vi "AutonControl.vi"(7 "Disabled":bool=TRUE, 8 "error in":errorcluster, 9 "Gamepad Data":T1, 10 "HMI to Control":T2, 11 "SensorInputData":T6) -> (0 "error out":errorcluster, 2 "HMI to Control Out":T2, 3 "SensorInputDataOut":T6)   [LabVIEW 2014]
uses:
  Typedefs/SensorInputData.ctl
  Typedefs/HMI_to_Control.ctl
  Typedefs/Arm States.ctl
  Typedefs/ClawStates.ctl
  Typedefs/IntakeWheelSenseOrManual.ctl
  Typedefs/GamepadData.ctl
  scriptlib/auto_data.vi
panel:
  out "autontime":i32
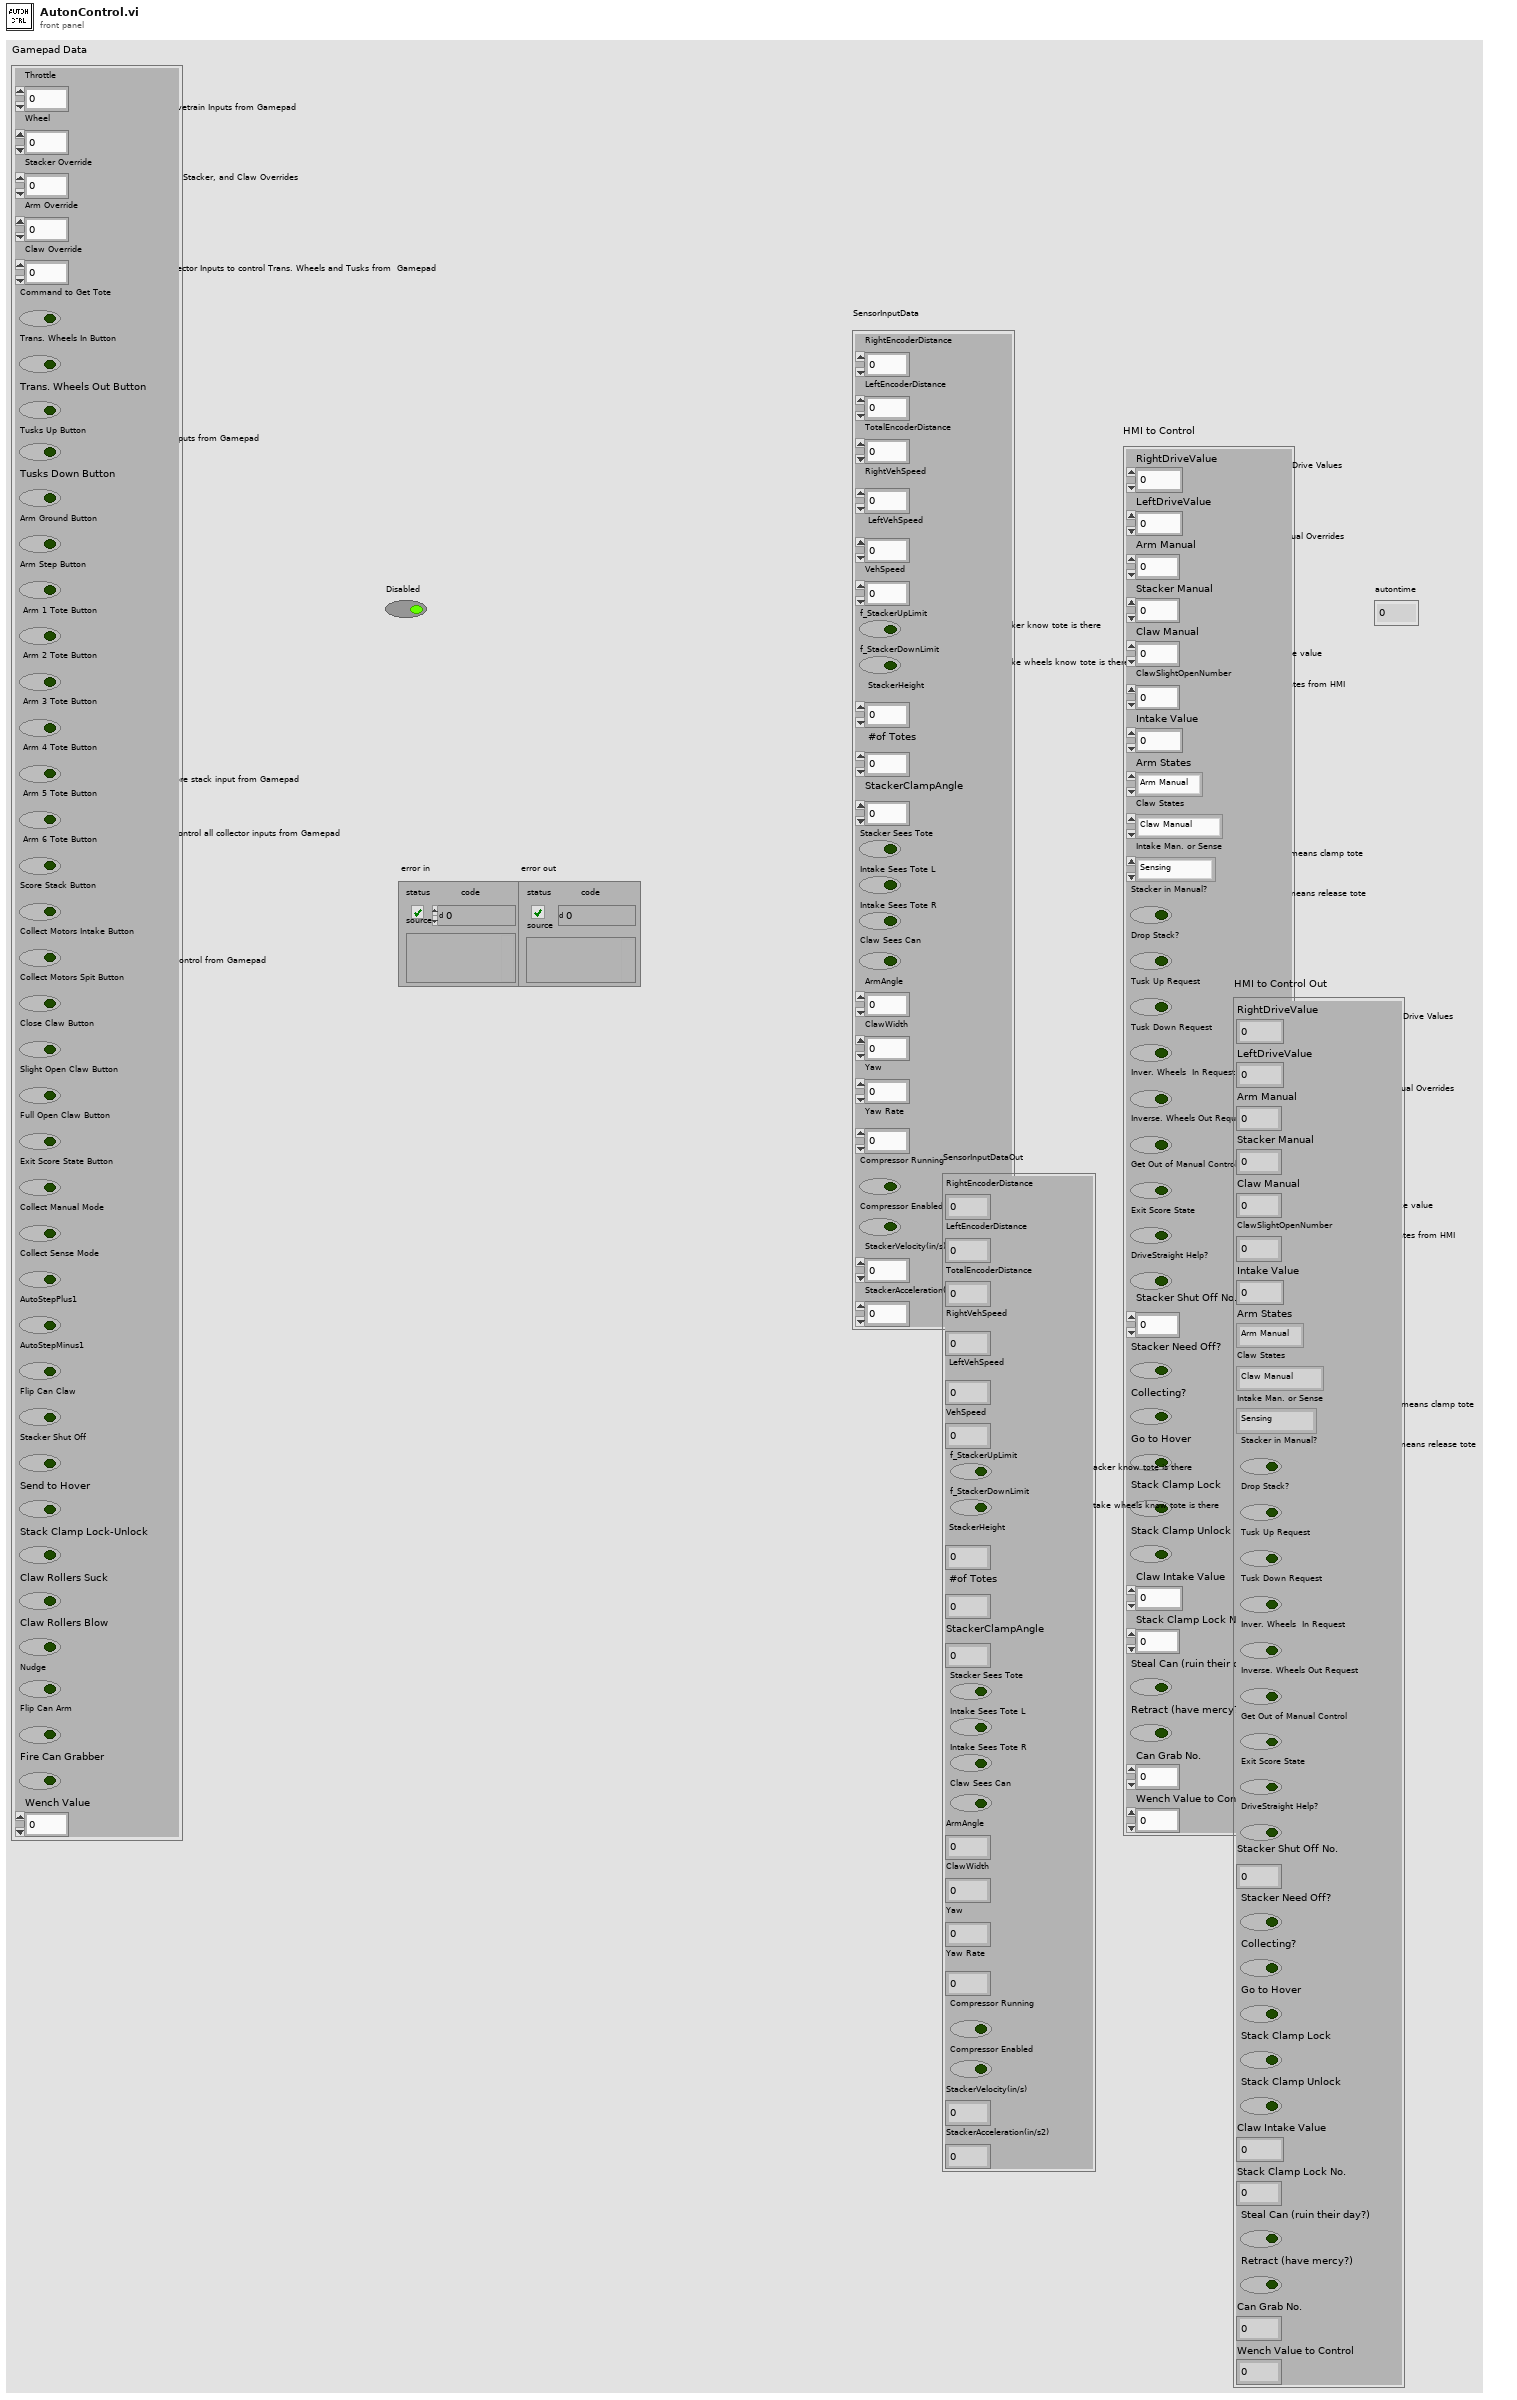
[diagram p1: front panel]
types:
  T1 = typedef "GamepadData.ctl" = cluster{"Throttle":dbl, "Wheel":dbl, "Stacker Override":dbl, "Arm Override ":dbl, "Claw Override":dbl, "Command to Get Tote":bool, "Trans. Wheels In Button":bool, "Trans. Wheels Out Button":bool, "Tusks Up Button":bool, "Tusks Down Button":bool, "Arm Ground Button":bool, "Arm Step Button":bool, " Arm 1 Tote Button":bool, " Arm 2 Tote Button":bool, " Arm 3 Tote Button ":bool, " Arm 4 Tote Button":bool, " Arm 5 Tote Button":bool, " Arm 6 Tote Button":bool, "Score Stack Button":bool, "Collect Motors Intake Button":bool, "Collect Motors Spit Button":bool, "Close Claw Button":bool, "Slight Open Claw Button":bool, "Full Open Claw Button ":bool, "Exit Score State Button":bool, "Collect Manual Mode ":bool, "Collect Sense Mode":bool, "AutoStepPlus1":bool, "AutoStepMinus1":bool, "Flip Can Claw":bool, "Stacker Shut Off":bool, "Send to Hover ":bool, "Stack Clamp Lock-Unlock ":bool, "Claw Rollers Suck ":bool, "Claw Rollers Blow ":bool, "Nudge":bool, "Flip Can Arm ":bool, "Fire Can Grabber":bool, "Wench Value":dbl}
  T2 = typedef "HMI_to_Control.ctl" = cluster{"RightDriveValue":dbl, "LeftDriveValue":dbl, "Arm Manual ":dbl, "Stacker Manual ":dbl, "Claw Manual ":dbl, "ClawSlightOpenNumber":i8, "Intake Value ":sgl, "Arm States":T3, "Claw States":T4, "Intake Man. or Sense":T5, "Stacker in Manual?":bool, "Drop Stack? ":bool, "Tusk Up Request":bool, "Tusk Down Request":bool, "Inver. Wheels  In Request":bool, "Inverse. Wheels Out Request ":bool, "Get Out of Manual Control":bool, "Exit Score State":bool, "DriveStraight Help?":bool, "Stacker Shut Off No.":i8, "Stacker Need Off?":bool, "Collecting?":bool, "Go to Hover":bool, "Stack Clamp Lock ":bool, "Stack Clamp Unlock ":bool, "Claw Intake Value ":sgl, "Stack Clamp Lock No. ":i8, "Steal Can (ruin their day?)":bool, "Retract (have mercy?)":bool, "Can Grab No. ":i8, "Wench Value to Control ":dbl}
  T3 = typedef "Arm States.ctl" = enum16{"Arm Manual ", "Ground", "Step", "1 Tote", "2 Tote", "3 Tote", "4 Tote", "5 Tote", "6 Tote", "Flip Can Arm", "Grab Can in auto", "Nudge"}
  T4 = typedef "ClawStates.ctl" = enum16{"Claw Manual ", "Claw Open", "Claw Closed", "Claw Slight Open", "Flip Can"}
  T5 = typedef "IntakeWheelSenseOrManual.ctl" = enum16{"Sensing", "Manual "}
  T6 = typedef "SensorInputData.ctl" = cluster{"RightEncoderDistance":dbl, "LeftEncoderDistance":dbl, "TotalEncoderDistance":dbl, "RightVehSpeed":dbl, "LeftVehSpeed":dbl, "VehSpeed":dbl, "f_StackerUpLimit":bool, "f_StackerDownLimit":bool, "StackerHeight":dbl, "#of Totes":u8, "StackerClampAngle":dbl, "Stacker Sees Tote":bool, "Intake Sees Tote L":bool, "Intake Sees Tote R":bool, "Claw Sees Can":bool, "ArmAngle":dbl, "ClawWidth":dbl, "Yaw":dbl, "Yaw Rate":dbl, "Compressor Running":bool, "Compressor Enabled":bool, "StackerVelocity(in/s)":dbl, "StackerAcceleration(in/s2)":dbl}
  T7 = typedef "vi_execute.ctl" = cluster{"arguments":string[], "command":string, "refnum valid check":bool, "vi_ind":u8}
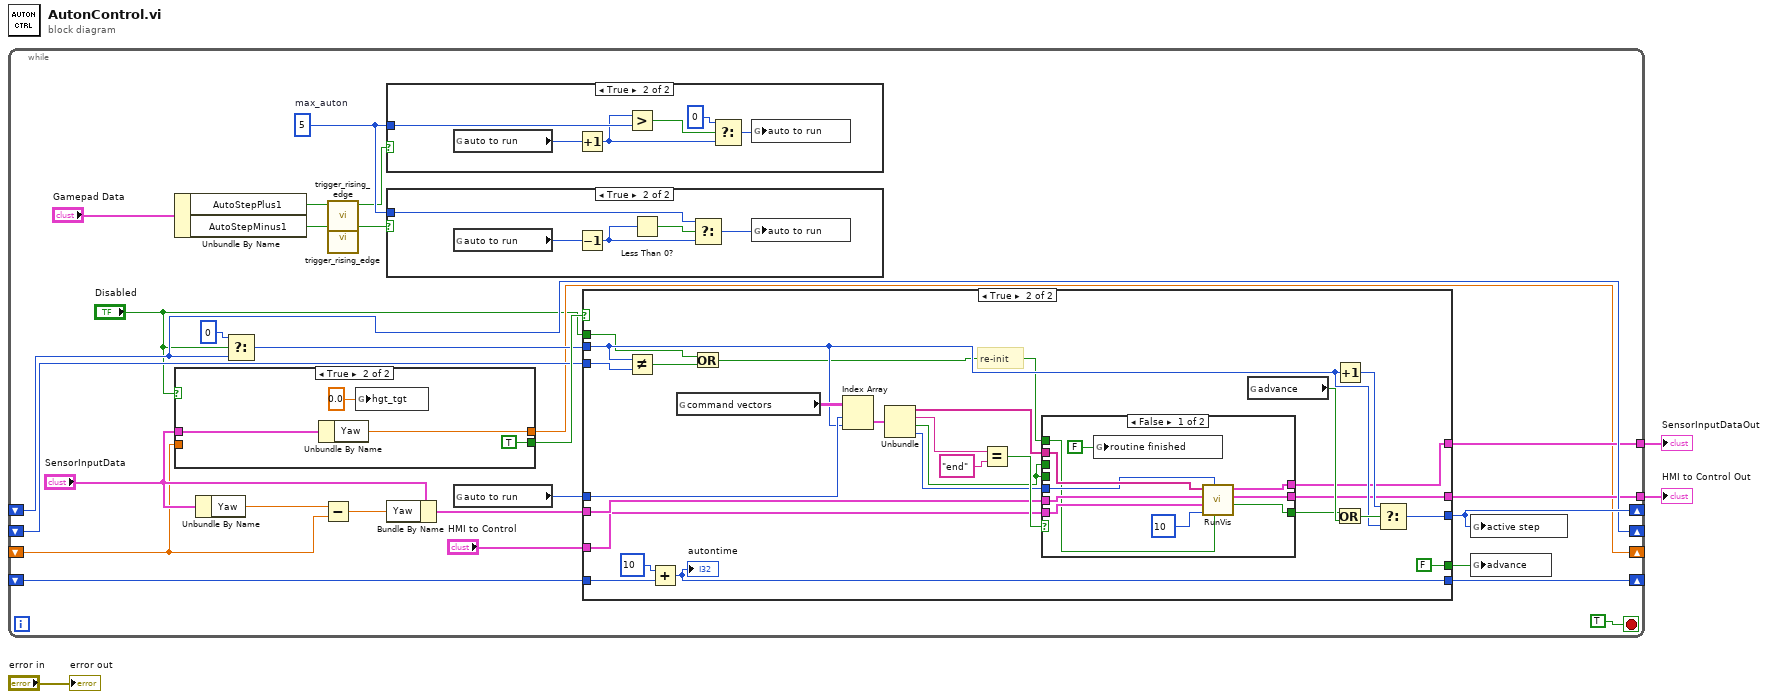
[diagram p0: block diagram]
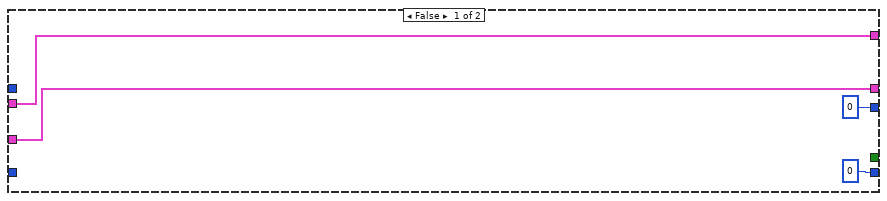
[diagram p4: hidden frame]
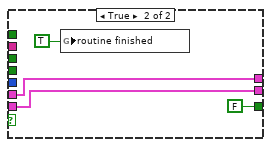
[diagram p5: hidden frame]
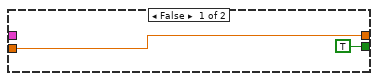
[diagram p6: hidden frame]
diagram:
  n1 = while {
    shift-right: [w26] -> _
    shift-left: _ -> [w25]
    shift-right: [w25] -> _
    shift-left: _ -> [w24]
    shift-right: [w21] -> _
    shift-left: _ -> [w20]
    tunnel: [w18] -> w2
    shift-right: [w16] -> _
    shift-left: _ -> [w11]
    tunnel: [w17] -> w1
    stop <- TRUE stop-if-true
    w9 = i8 5  # max_auton
    n2 = Unbundle By Name("Gamepad Data") -> ("AutoStepPlus1"=w8:bool, "AutoStepMinus1"=w6:bool)
    n3 = case shown="True" "Disabled" {
      tunnel: [TRUE ("init_done") TRUE ("init_done")] -> w30
      tunnel: "SensorInputData" -> [_ w90]
      tunnel: [w87 w89] -> w16
      tunnel: w11 -> [w87 _]
      frame False {
      }
      frame True {
        n4 = Unbundle By Name(w90) -> ("Yaw"=w89:dbl)
        n5 = global write "auto_data.vi" "hgt_tgt"(0.0 ("hgt_tgt")) -> ()
      }
    }
    n6 = Unbundle By Name("SensorInputData") -> ("Yaw"=w13:dbl)
    n7 = Select(t=0, s="Disabled", f=w25) -> (s? t:f=w27:i32)
    n8 = Subtract(x=w13, y=w11) -> (x-y=w12:dbl)
    n9 = call "trigger_rising_edge.vi"("input"=w8) -> ("rising"=w7:bool)  [unwired: 10 in]
    n10 = call "trigger_rising_edge.vi"("input"=w6) -> ("rising"=w5:bool)  [unwired: 10 in]
    n11 = case shown="True" w7 {
      tunnel: w9 -> [_ w39]
      frame False {
      }
      frame True {
        n12 = global read "auto_data.vi" "auto to run"() -> (w41:i8)
        n13 = Increment(x=w41) -> (x+1=w38:i8)
        n14 = Greater?(x=w38, y=w39) -> (0:w40:bool)
        n15 = Select(t=i8 0, s=w40, f=w38) -> (s? t:f=w36:i8)
        n16 = global write "auto_data.vi" "auto to run"(w36) -> ()
      }
    }
    n17 = case shown="True" w5 {
      tunnel: w9 -> [_ w32]
      frame False {
      }
      frame True {
        n18 = global read "auto_data.vi" "auto to run"() -> (w35:i8)
        n19 = Decrement(x=w35) -> (x-1=w31:i8)
        n20 = Less Than 0?(x=w31) -> (x < 0?=w34:bool)
        n21 = Select(t=w32, s=w34, f=w31) -> (s? t:f=w33:i8)
        n22 = global write "auto_data.vi" "auto to run"(w33) -> ()
      }
    }
    n23 = Bundle By Name(cluster="SensorInputData", "Yaw"=w12) -> (w15:T6)
    n24 = global read "auto_data.vi" "auto to run"() -> (w29:i8)
    n25 = case shown="True" w30 {
      tunnel: w29 -> [_ w62]
      tunnel: w27 -> [_ w61]
      tunnel: [0 w63] -> w26
      tunnel: w24 -> [_ w60]
      tunnel: [_ FALSE ("advance")] -> w23
      tunnel: [0 w57] -> w21
      tunnel: w20 -> [_ w56]
      tunnel: w15 -> [w45 w55]
      tunnel: "HMI to Control" -> [w44 w54]
      tunnel: [w45 w52] -> w18
      tunnel: [w44 w51] -> w17
      tunnel: "Disabled" -> [_ w46]
      frame False {
      }
      frame True {
        # "re-init"
        n26 = Not Equal?(x=w61, y=w60) -> (x != y?=w48:bool)
        n27 = Add(x=10, y=w56) -> (x+y=w57:i32)
        "autontime" <- w57
        n28 = global read "auto_data.vi" "command vectors"() -> (w72:T7[][])
        n29 = Or(x=w46, y=w48) -> (x .or. y?=w47:bool)
        n30 = Index Array(array=w72, index (row)=w62, index (col)=w61) -> (element=w71:T7)
        n31 = Unbundle(w71) -> ("arguments"=w70:string[], "command"=w69:string, "refnum valid check"=w49:bool, "vi_ind"=w53:u8)
        n32 = Equal?(x=w69, y="end") -> (x = y?=w67:bool)
        n33 = case shown="False" w67 {
          tunnel: w70 -> [w79 _]
          tunnel: w55 -> [w81 w84]
          tunnel: w54 -> [w80 w83]
          tunnel: w53 -> [w78 _]
          tunnel: w47 -> [w76 _]
          tunnel: [w75 w84] -> w52
          tunnel: [w74 w83] -> w51
          tunnel: [w73 FALSE ("Done")] -> w50
          tunnel: w49 -> [_ _]
          tunnel: w49 -> [_ _]
          frame False {
            n34 = global write "auto_data.vi" "routine finished"(FALSE ("routine finished")) -> ()
            n35 = call "RunVis.vi"("Re-Init"=w76, "Index"=w78, "dt"=i8 10, "HMI to Control"=w80, "SensorInputData"=w81, "arguments"=w79) -> ("Done"=w73:bool, "HMI to Control Out"=w74:T2, "SensorInputDataOut"=w75:T6)  [unwired: 3 in]
          }
          frame True {
            n36 = global write "auto_data.vi" "routine finished"(TRUE ("routine finished")) -> ()
          }
        }
        n37 = global read "auto_data.vi" "advance"() -> (w66:bool)
        n38 = Increment(x=w61) -> (x+1=w64:i32)
        n39 = Or(x=w50, y=w66) -> (x .or. y?=w65:bool)
        n40 = Select(t=w64, s=w65, f=w61) -> (s? t:f=w63:i32)
      }
    }
    n41 = global write "auto_data.vi" "active step"(w26) -> ()
    n42 = global write "auto_data.vi" "advance"(w23) -> ()
  }
  "SensorInputDataOut" <- w2
  "HMI to Control Out" <- w1
  "error out" <- "error in"
